vi "Get Actor Self Enqueuer.vi"(11 "Actor in":refnum<class "Actor.lvclass">) -> (3 "Self Enqueuer":refnum<class "Message Enqueuer.lvclass">)   [LabVIEW 2020, in "Utility.lvlib" / "Private Actor.lvclass"]
uses:
  Private Actor.lvclass
  PPL/HDH.Actor Framework.Core.Actor.lvlibp/1abvi3w/vi.lib/ActorFramework/Actor/Actor.lvclass
  PPL/HDH.Actor Framework.Core.Actor.lvlibp/1abvi3w/vi.lib/ActorFramework/Message Enqueuer/Message Enqueuer.lvclass
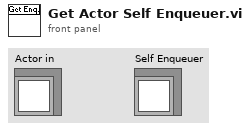
[diagram p1: front panel]
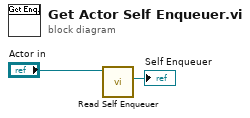
[diagram p0: block diagram]
diagram:
  n1 = call "Read Self Enqueuer.vi"("Actor"="Actor in") -> ("Self Enqueuer"=→"Self Enqueuer":refnum<class "Message Enqueuer.lvclass">)  [unwired: 10 in]
